vi "1553 BM - Read the Queue Modified.vi"(8 "Error In (none)":errorcluster, 10 "BIU Number (1)":u8=1, 11 "Module Handle":u32) -> (0 "Error Out":errorcluster, 2 "Short Queue Entry":T1, 3 "ModuleHandle Out":u32, 5 "Queue Entry full":bool)   [LabVIEW 2020, in "AIM MIL-STD-1553 Hardware API.lvlib"]
doc: "<B>ApiCmdQueueRead</B>\n\nThis function is used to read a single 1553 message structure from the head of the BM monitor buffer queue. If the queue is empty the function returns the queue empty error. If the queue has overflowed the function returns an overflow error. After an overflow has occured, the queueing system must be stopped and restarted again with the 1553 BM - Queue Stop and then the 1553 BM - Initialize Record with Queuing Mode / 1553 BM - Flush the Queue functions. The internal queue pointer is incremented automatically such that subsequent calls to this function can be made and will return the next entry.\n\n<B>Input Parameters:</B>\n\nModule Handle - Reference to the device as obtained from a call to: 1553 General - Obtain a Device Reference.vi\n\nBIU Number (1) - BIU number (one-based) of the bus interface unit.\n\n<B> Output Parameters: </B>\n\nTime Stamp - The time at which the queue entry was made.\n\nTransmit RT Status Word - The status of the transmitting RT. Only valid for RT->RT transfers.\n\nReceive RT Status Word - The status of the receiving RT.\n\nQueue Entry\n\nRT Address - The address of the receiving RT.\nSub-address - The sub-address of the receiving RT (or mode code in numeric form).\nMode code - The mode code.\nDirection - The direction of the transfer (receive, transmit).\nType - The type of transfer (sub-address, mode code).\n\nFor RT->RT Transfers:\n\nRT Address 2 - The address of the transmitting RT.\nSub-address 2 - The sub-address of the transmitting RT (or mode code in numeric form).\nMode code 2 - The mode code.\nDirection 2 - The direction of the transfer (receive, transmit).\nType 2 - The type of transfer (sub-address, mode code).\n\nWord Count - The data word count associated with the transfer.\nBus - The bus along which the transfer was sent (primary, secondary)."
uses:
  AIM MIL-STD-1553 Hardware API.lvlib
  Shortened Queue Entry.ctl
  <instrlib>/_AIM MIL-STD-1553/PCI-1553 Release/LS-Utility/1553 Utility - DLL Path Global.vi
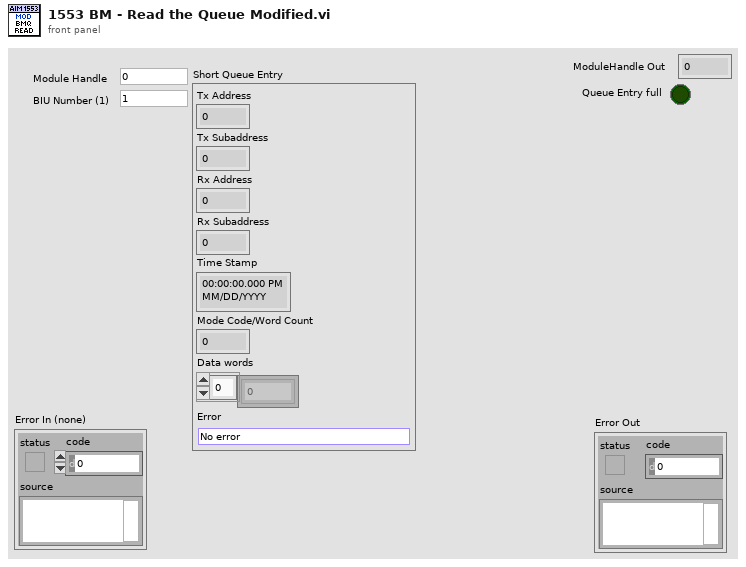
[diagram p1: front panel]
types:
  T1 = typedef "AIM MIL-STD-1553 Hardware API.lvlib/Shortened Queue Entry.ctl" = cluster{"Tx Address":u8, "Tx Subaddress":u8, "Rx Address":u8, "Rx Subaddress":u8, "Time Stamp":timestamp, "Mode Code/Word Count":u8, "Data words":u16[], "Error ":enum16{"No error", "Terminal no response error", "Manchester coding error", "High bit count error", "Low bit count error", "Parity error", "Inverted sync error", "Interw ord gap error", "Transmission on both MILbus channels", "Reserved mode code error", "Early response or gap too short", "ME bit set in status word", "Status word exception error", "High wordcount error", "Low wordcount error", "Illegal command word"}}
  T2 = enum16{"No error", "Terminal no response error", "Manchester coding error", "High bit count error", "Low bit count error", "Parity error", "Inverted sync error", "Interw ord gap error", "Transmission on both MILbus channels", "Reserved mode code error", "Early response or gap too short", "ME bit set in status word", "Status word exception error", "High wordcount error", "Low wordcount error", "Illegal command word"}
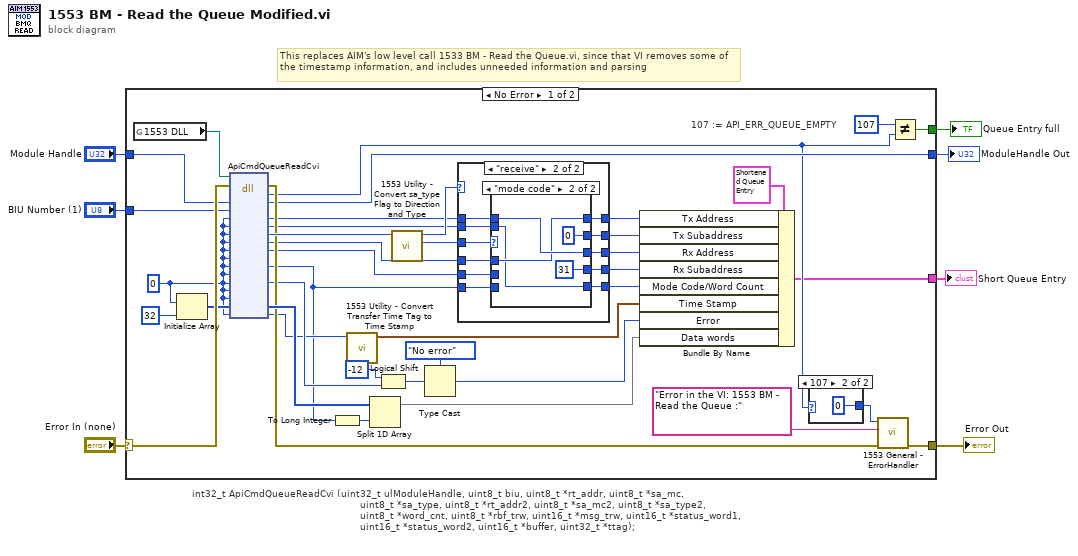
[diagram p0: block diagram]
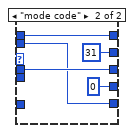
[diagram p3: hidden frame]
diagram:
  # "This replaces AIM's low level call 1533 BM - Read the Queue.vi, since that VI removes some of the timestamp information, and includes unneeded information and parsing"
  # "int32_t ApiCmdQueueReadCvi (uint32_t ulModuleHandle, uint8_t biu, uint8_t *rt_addr, uint8_t *sa_mc, \n                                                        uint8_t *sa_type, uint8_t *rt_addr2, uint8_t *sa_mc2, uint8_t *sa_type2, \n                                                        uint8_t *word_cnt, uint8_t *rbf_trw, uint16_t *msg_trw, uint16_t *status_word1, \n                                                        uint16_t *status_word2, uint16_t *buffer, uint32_t *ttag);"
  n1 = case shown="No Error" "Error In (none)" {
    selector: "Error In (none)" -> [w47 w93]
    tunnel: [w39 w93] -> w6
    tunnel: "Module Handle" -> [w46 w92]
    tunnel: "BIU Number (1)" -> [w45 _]
    tunnel: [w36 w92] -> w3
    tunnel: [w31 _] -> w2
    tunnel: [w23 _] -> w1
    frame No Error {
      w11 = u8 0 ("rt_addr")
      # "107 := API_ERR_QUEUE_EMPTY"
      n2 = global read "1553 Utility - DLL Path Global.vi" "1553 DLL"() -> (w40:path)
      n3 = Initialize Array(w11, 32 ("dimension size")) -> (w43:u8[])
      n4 = dll-call lib="C:/Program Files/AIM GmbH/PCI-1553-WINDOWS-V1120/LabView/api_mil.dll" fn="ApiCmdQueueReadCvi"(path in=w40, error in=w47, "ulModuleHandle"=w46, "biu"=w45, "rt_addr"=w11, "sa_mc"=w11, "sa_type"=w11, "rt_addr2"=w11, "sa_mc2"=w11, "sa_type2"=w11, "word_cnt"=w11, "rbf_trw"=w11, "msg_trw"=w11, "status_word1"=w11, "status_word2"=w11, "buffer"=w43, "ttag"=w11) -> (error out=w38:errorcluster, "err"=w30:i32, "ulModuleHandle"=w36:u32, "rt_addr"=w21:u8, "sa_mc"=w20:u8, "sa_type"=w42:u8, "rt_addr2"=w19:u8, "sa_mc2"=w18:u8, "word_cnt"=w9:u8, "msg_trw"=w28:u16, "buffer"=w41:u16[], "ttag"=w26:u32)  [unwired: 2 in, 5 out]
      n5 = To Long Integer(number=w9) -> (32bit integer=w34:i32)
      n6 = call <instrlib>:"1553 Utility - Convert Transfer Time Tag to Time Stamp.vi"("Transfer Time Tag"=w26) -> ("Time Stamp"=w10:timestamp)  [unwired: 10 in]
      n7 = Split 1D Array(array=w41, index=w34) -> (first subarray=w13:u16[])  [unwired: 1 out]
      n8 = Logical Shift(y=i16 -12, x=w28) -> (x << y=w29:u16)
      n9 = call <instrlib>:"1553 Utility - Convert sa_type Flag to Direction and Type.vi"("sa_type flag (0)"=w42) -> ("Type"=w12:enum16{"sub-address", "mode code"}, "Direction"=w22:enum16{"receive", "transmit"})  [unwired: 9 in]
      n10 = Type Cast(type=T2."No error" ("Error"), x=w29) -> (*(type *) &x=w24:T2)
      n11 = case shown="\"receive\"" w22 {
        tunnel: w21 -> [w57 w79]
        tunnel: w20 -> [w55 w77]
        tunnel: w19 -> [w53 w75]
        tunnel: w18 -> [w51 w73]
        tunnel: [w56 w78] -> w17
        tunnel: [w54 w76] -> w16
        tunnel: [w52 w74] -> w15
        tunnel: [w50 w72] -> w14
        tunnel: w12 -> [w58 w69]
        tunnel: w9 -> [w49 w71]
        tunnel: [w48 w70] -> w8
        frame "transmit" {
          n12 = case shown="\"sub-address\", Default" w58 {
            tunnel: w57 -> [w63 w68]
            tunnel: [w63 w68] -> w56
            tunnel: w55 -> [w62 w64]
            tunnel: [w62 u8 31 ("sa_mc")] -> w54
            tunnel: w53 -> [w61 w66]
            tunnel: [w61 w66] -> w52
            tunnel: w51 -> [w60 _]
            tunnel: [w60 u8 0 ("sa_mc")] -> w50
            tunnel: w49 -> [w59 _]
            tunnel: [w59 w64] -> w48
            frame "sub-address", Default {
            }
            frame "mode code" {
            }
          }
        }
        frame "receive" {
          n13 = case shown="\"mode code\"" w69 {
            tunnel: w79 -> [w83 w87]
            tunnel: [w81 w86] -> w78
            tunnel: w77 -> [w82 w85]
            tunnel: [w80 u8 0 ("sa_mc")] -> w76
            tunnel: w75 -> [w81 w86]
            tunnel: [w83 w87] -> w74
            tunnel: w73 -> [w80 _]
            tunnel: [w82 u8 31 ("sa_mc")] -> w72
            tunnel: w71 -> [w84 _]
            tunnel: [w84 w85] -> w70
            frame "sub-address", Default {
            }
            frame "mode code" {
            }
          }
        }
      }
      n14 = Bundle By Name(cluster=T1 {"Tx Address"=0, "Tx Subaddress"=0, "Rx Address"=0, "Rx Subaddress"=0, "Time Stamp"=timestamp(0 s since 1904-01-01), "Mode Code/Word Count"=0, "Data words"=[], "Error "=enum."No error"} ("Short Queue Entry"), "Tx Address"=w17, "Tx Subaddress"=w16, "Rx Address"=w15, "Rx Subaddress"=w14, "Mode Code/Word Count"=w8, "Time Stamp"=w10, "Error"=w24, "Data words"=w13) -> (w23:T1)
      n15 = case shown="107" w30 {
        selector: w30 -> [w90 _]
        tunnel: [w90 0] -> w35
        frame 0, Default {
        }
        frame 107 {
        }
      }
      n16 = call <instrlib>:"1553 General - ErrorHandler.vi"("error in (no error)"=w38, "Additionally Error Information"="Error in the VI: 1553 BM - Read the Queue :" ("source"), "AIM Error Code"=w35) -> ("error out"=w39:errorcluster)  [unwired: 8 in]
      n17 = Not Equal?(x=107, y=w30) -> (x != y?=w31:bool)
    }
    frame Error {
    }
  }
  "Error Out" <- w6
  "ModuleHandle Out" <- w3
  "Queue Entry full" <- w2
  "Short Queue Entry" <- w1
